vi "LabVIEW REST Examples.vi"   [LabVIEW 2021]
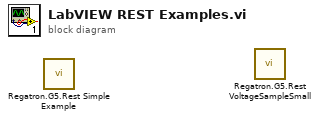
[diagram p0: block diagram]
diagram:
  n1 = call "Regatron.G5.Rest Simple Example.vi"() -> ()  [unwired: 12 in]
  n2 = call "Regatron.G5.Rest VoltageSampleSmall.vi"() -> ()  [unwired: 12 in]
